vi "get supported channel classifications.vi"(8 "error in":errorcluster, 11 "module configuration in":refnum<class "shared memory configuration.lvclass">) -> (0 "error out":errorcluster, 2 "supported types":T1[](array[typedef]), 3 "module configuration out":refnum<class "shared memory configuration.lvclass">)   [LabVIEW 2013, in "shared memory configuration.lvclass"]
doc: "Provides an interface for determining the channel types supported by a given configuration/runtime class pairing. This should be overridden by a child class in order to allow for improved validation of a given configuration."
uses:
  shared memory configuration.lvclass
  <vilib>/NI/Tag Bus Module Framework/channel/channel classification.ctl
  <vilib>/NI/Tag Bus Module Framework/channel/TBM channel.lvclass
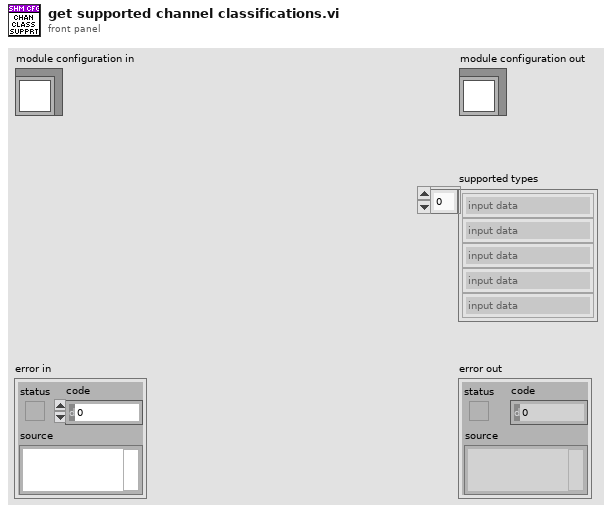
[diagram p1: front panel]
types:
  T1 = typedef "TBM channel.lvclass/channel classification.ctl" = enum16{"input data", "output data", "processing parameter", "processing result"}
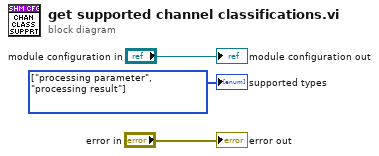
[diagram p0: block diagram]
diagram:
  w1 = T1[] [enum."processing parameter", enum."processing result"] items=["input data", "output data", "processing parameter", "processing result"] ("supported types")
  "error out" <- "error in"
  "module configuration out" <- "module configuration in"
  "supported types" <- w1
